vi "Close_Actor_Test.vi"(8 "error in (no error)":errorcluster caption="entrée d'erreur (pas d'erreur)", 11 "Test (Default) en entrée":refnum<class "Actor Test Firebase.lvclass">) -> (0 "error out":errorcluster caption="sortie d'erreur", 3 "Test (Default) en sortie":refnum<class "Actor Test Firebase.lvclass">)   [LabVIEW 2020, in "Library Core.lvlib" / "Actor Test Firebase.lvclass"]
uses:
  Actor Test Firebase.lvclass
  Actor Test (Default)/Actor Test (Default).lvclass
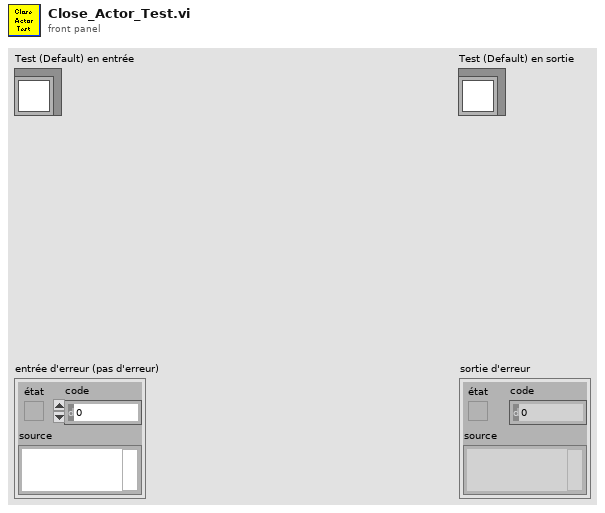
[diagram p1: front panel]
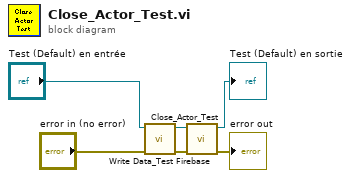
[diagram p0: block diagram]
diagram:
  n1 = call-dynamic "Write Data_Test Firebase.vi"("error in (no error)"="error in (no error)", "Actor Test Firebase en entrée"="Test (Default) en entrée") -> ("error out"=w3:errorcluster, "Actor Test Firebase en sortie"=w4:refnum<class "Actor Test Firebase.lvclass">)  [unwired: 8 in]
  n2 = call-parent "Close_Actor_Test.vi"("error in (no error)"=w3, "Test (Default) en entrée"=w4) -> ("error out"=→"error out":errorcluster, "Test (Default) en sortie"=→"Test (Default) en sortie":refnum<class "Actor Test Firebase.lvclass">)  [unwired: 8 in]
